vi "质控配样.vi"() -> ()   [LabVIEW 2016, in "质控单元V4.lvlib"]
panel:
  in  "Tab Control 5":enum32{"参数"}(tab)
  out "剩余时间":string
  out "当前步骤":string
  out "当前流程":string
  out "告警状态":string
  out "液位状态":string
  out "运行状态":string
  out "通讯状态":bool caption="状态"
  in  "Tab Control 4":enum32{"参数"}(tab)
  in  "停止":bool
  in  "目标浓度(mg/L)":sgl
  in  "标样浓度(mg/L)":sgl
  in  "启动":bool
  in  "请选择模块":T1(radio)=enum."氨氮"
  # "仪器状态"
  # "参数设置"
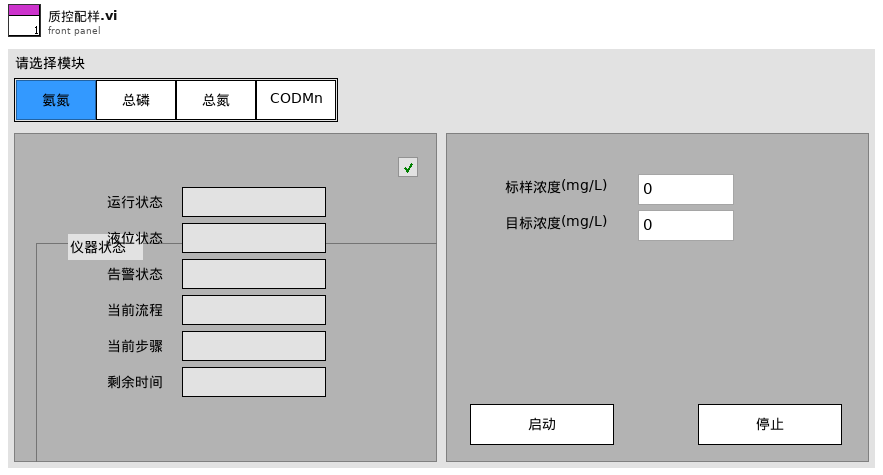
[diagram p1: front panel]
types:
  T1 = enum32{"未选择", "氨氮", "总磷", "总氮", "CODMn", "CODCr", "氟化物", "挥发酚"}
  T2 = cluster{"氨氮":bool, "总磷":bool, "总氮":bool, "CODMn":bool, "CODCr":bool, "氟化物":bool, "挥发酚":bool}
  T3 = typedef "质控单元V4.lvlib/质控slave id.ctl" = enum16{"null", "氨氮", "总磷", "总氮", "CODMn", "CODCr", "氟化物", "挥发酚"}
  T4 = typedef "质控单元V4.lvlib/质控流程控制.ctl" = enum16{"待机", "启动进样流程", "启动加标流程", "启动排液流程", "启动水样润洗流程", "启动加标润洗流程", "停止流程"}
  T5 = typedef "质控单元V4.lvlib/质控仪器状态显示.ctl" = cluster{"运行模式":string, "运行状态":string, "液位状态":string, "告警状态":string, "当前流程":string, "当前步骤":string, "剩余时间":string}
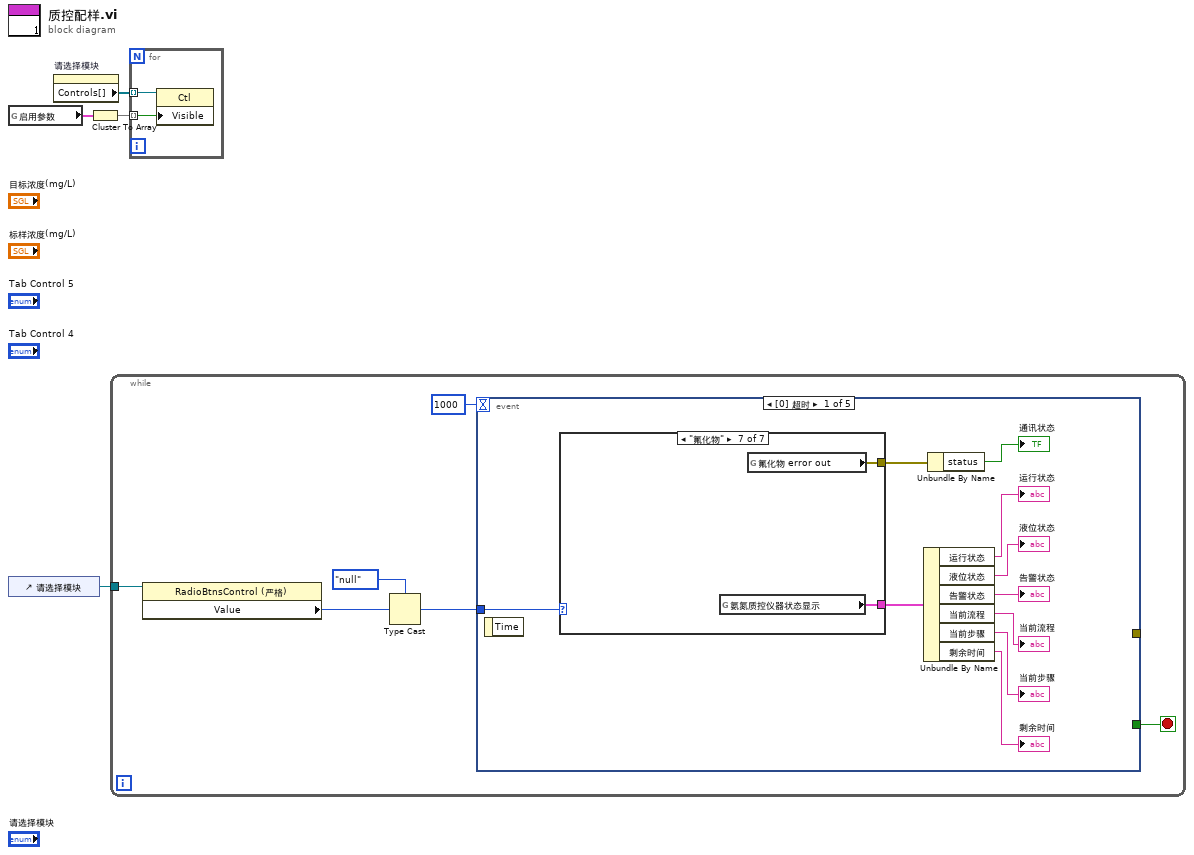
[diagram p0: block diagram]
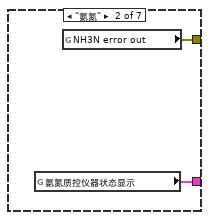
[diagram p3: hidden frame]
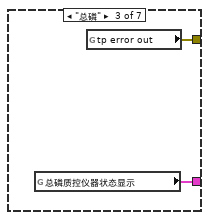
[diagram p4: hidden frame]
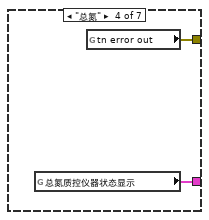
[diagram p5: hidden frame]
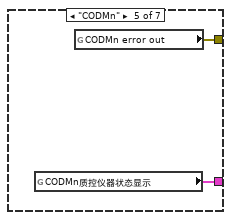
[diagram p6: hidden frame]
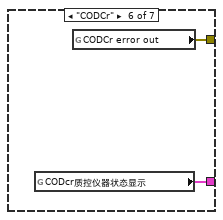
[diagram p7: hidden frame]
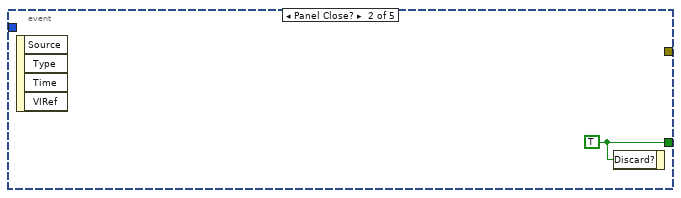
[diagram p8: hidden frame]
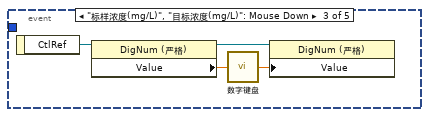
[diagram p9: hidden frame]
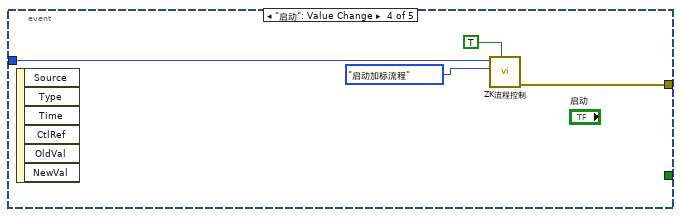
[diagram p10: hidden frame]
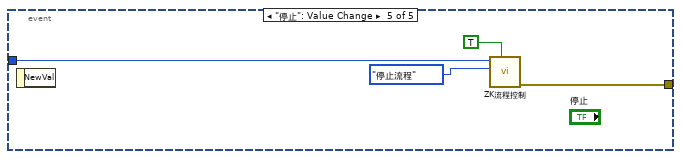
[diagram p11: hidden frame]
diagram:
  n1 = global read "ZK断电保存全局变量.vi" "启用参数"() -> (w4:T2)
  n2 = control-ref of="请选择模块"() -> (w1:refnum<vi>)
  n3 = property on="请选择模块" class="RadioBtnsControl (严格)"() -> ("Controls[]"=w3:refnum<vi>[])  [unwired: 2 in, 2 out]
  n4 = Cluster To Array(cluster=w4) -> (array=w2:bool[])
  n5 = while {
    tunnel: w1 -> [w6]
    stop <- w10 stop-if-true
    n6 = property class="RadioBtnsControl (严格)"(reference=w6) -> ("Value"=w8:T1)  [unwired: 1 in, 2 out]
    n7 = Type Cast(type=质控slave_id."null" ("请选择模块"), x=w8) -> (*(type *) &x=w5:T3)
    n8 = event shown="[0] 超时" {
      selector: _ -> [_ _ _ _ _]
      dyn-events: _ -> [_ _ _ _ _]
      timeout: 1000 -> [_ _ _ _ _]
      tunnel: [_ w33 _ _ _] -> w10
      tunnel: [_ _ _ w39 w43] -> _
      tunnel: w5 -> [w18 _ _ w38 w42]
      event Timeout {
        n9 = event-data() -> ()  [unwired: 1 in, 1 out]
        n10 = case shown="\"氟化物\"" w18 {
          tunnel: [_ w22 w24 w26 w28 w30 w32] -> w20
          tunnel: [_ w21 w23 w25 w27 w29 w31] -> w19
          frame "null", Default {
          }
          frame "氨氮" {
            n11 = global read "ZK非断电保存全局变量.vi" "氨氮质控仪器状态显示"() -> (w22:T5)
            n12 = global read "ZK非断电保存全局变量.vi" "NH3N error out"() -> (w21:errorcluster)
          }
          frame "总磷" {
            n13 = global read "ZK非断电保存全局变量.vi" "总磷质控仪器状态显示"() -> (w24:T5)
            n14 = global read "ZK非断电保存全局变量.vi" "tp error out"() -> (w23:errorcluster)
          }
          frame "总氮" {
            n15 = global read "ZK非断电保存全局变量.vi" "总氮质控仪器状态显示"() -> (w26:T5)
            n16 = global read "ZK非断电保存全局变量.vi" "tn error out"() -> (w25:errorcluster)
          }
          frame "CODMn" {
            n17 = global read "ZK非断电保存全局变量.vi" "CODMn质控仪器状态显示"() -> (w28:T5)
            n18 = global read "ZK非断电保存全局变量.vi" "CODMn error out"() -> (w27:errorcluster)
          }
          frame "CODCr" {
            n19 = global read "ZK非断电保存全局变量.vi" "CODcr质控仪器状态显示"() -> (w30:T5)
            n20 = global read "ZK非断电保存全局变量.vi" "CODCr error out"() -> (w29:errorcluster)
          }
          frame "氟化物" {
            n21 = global read "ZK非断电保存全局变量.vi" "氨氮质控仪器状态显示"() -> (w32:T5)
            n22 = global read "ZK非断电保存全局变量.vi" "氟化物 error out"() -> (w31:errorcluster)
          }
        }
        n23 = Unbundle By Name(w20) -> ("运行状态"=→"运行状态":string, "液位状态"=→"液位状态":string, "告警状态"=→"告警状态":string, "当前流程"=→"当前流程":string, "当前步骤"=→"当前步骤":string, "剩余时间"=→"剩余时间":string)
        n24 = Unbundle By Name(w19) -> ("status"=→"通讯状态":bool)
      }
      event Panel Close? {
        w33 = TRUE ("放弃？")
        n25 = event-data() -> ()  [unwired: 1 in, 4 out]
        n26 = event-data("Discard?"=w33) -> ()  [unwired: 1 in, 1 out]
      }
      event "标样浓度(mg/L)", "目标浓度(mg/L)": Mouse Down {
        n27 = event-data() -> ("CtlRef"=w37:refnum<vi>)  [unwired: 1 in]
        n28 = property class="DigNum (严格)"(reference=w37) -> (reference out=w36:refnum<vi>, "Value"=w35:sgl)  [unwired: 1 in, 1 out]
        n29 = call "数字键盘.vi"("OldNumber"=w35) -> ("NewNumber"=w34:sgl)
        n30 = property class="DigNum (严格)"(reference=w36, "Value"=w34) -> ()  [unwired: 1 in, 2 out]
      }
      event "启动": Value Change {
        n31 = event-data() -> ()  [unwired: 1 in, 6 out]
        n32 = call "ZK流程控制.vi"("是否启用通讯通知"=TRUE, "流程控制"=质控流程控制."启动加标流程", "Slave ID"=w38) -> ("error out"=w39:errorcluster)  [unwired: 8 in]
      }
      event "停止": Value Change {
        n33 = event-data() -> ()  [unwired: 1 in, 1 out]
        n34 = call "ZK流程控制.vi"("是否启用通讯通知"=TRUE, "流程控制"=质控流程控制."停止流程", "Slave ID"=w42) -> ("error out"=w43:errorcluster)  [unwired: 8 in]
      }
    }
  }
  n35 = for {
    tunnel: w3 -> [w47] mode=indexing
    tunnel: w2 -> [w46] mode=indexing
    n36 = property class="Ctl"(reference=w47, "Visible"=w46) -> ()  [unwired: 1 in, 2 out]
  }
